vi "Q5.vi"() -> ()   [LabVIEW 2020]
uses:
  <vilib>/Utility/file.llb/Read Delimited Spreadsheet (DBL).vi
panel:
  out "Conversion Factor":dbl
  in  "file path (dialog if empty)":path
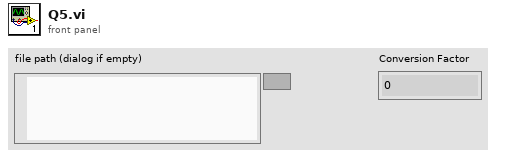
[diagram p1: front panel]
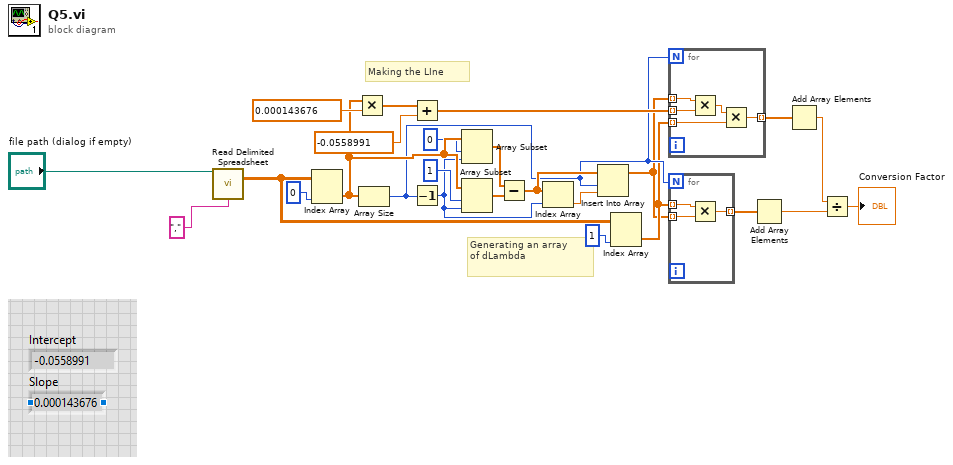
[diagram p0: block diagram]
diagram:
  # "Generating an array\nof dLambda"
  # "Making the LIne"
  n1 = call-poly <vilib>:"Read Delimited Spreadsheet.vi"("file path (dialog if empty)"="file path (dialog if empty)", "delimiter (\\t)"="," ("delimiter (\\t)")) -> ("all rows"=w23:dbl[][])  [unwired: 8 in, 5 out]
  n2 = Index Array(array=w23, index (col)=0 ("disabled index (col)")) -> (element=w16:dbl[])  [unwired: 1 in]
  n3 = Multiply(x=w16, y=0.000143676) -> (x*y=w20:dbl[])
  n4 = Array Size(array=w16) -> (size(s)=w7:i32)
  n5 = Add(x=w20, y=-0.0558991) -> (x+y=w17:dbl[])
  n6 = Decrement(x=w7) -> (x-1=w11:i32)
  n7 = Array Subset(array=w16, index=0, length=w11) -> (w12:dbl[])
  n8 = Array Subset(array=w16, index=1, length=w11) -> (w13:dbl[])
  n9 = Subtract(x=w12, y=w13) -> (x-y=w9:dbl[])
  n10 = Index Array(array=w9, index=w11) -> (element=w10:dbl)
  n11 = Insert Into Array(array=w9, index=w7, new element=w10) -> (w5:dbl[])
  n12 = Index Array(array=w23, index (col)=1 ("disabled index (col)")) -> (element=w6:dbl[])  [unwired: 1 in]
  n13 = for {
    N: w7 -> [_]
    tunnel: w17 -> [w29] mode=indexing
    tunnel: w5 -> [w30] mode=indexing
    tunnel: w6 -> [w27] mode=indexing
    tunnel: [w26] -> w8 mode=indexing
    n14 = Multiply(x=w30, y=w29) -> (x*y=w28:dbl)
    n15 = Multiply(x=w28, y=w27) -> (x*y=w26:dbl)
  }
  n16 = for {
    N: w7 -> [_]
    tunnel: w6 -> [w33] mode=indexing
    tunnel: w5 -> [w32] mode=indexing
    tunnel: [w31] -> w4 mode=indexing
    n17 = Multiply(x=w33, y=w32) -> (x*y=w31:dbl)
  }
  n18 = Add Array Elements(numeric array=w4) -> (sum=w2:dbl)
  n19 = Add Array Elements(numeric array=w8) -> (sum=w3:dbl)
  n20 = Divide(x=w3, y=w2) -> (x/y=→"Conversion Factor":dbl)
